vi "Drying_Process (SubVI).vi"(9 "Array 2":string[](array[string]), 10 "reference in":refnum<vi>, 11 "Array in":refnum<vi>) -> (1 "Array":string[](array[string]), 2 "Boolean":bool, 3 "empty?":bool)   [LabVIEW 2019]
uses:
  <vilib>/numeric/Random Number (Range) DBL.vi
  16b95fc4-76d9-4825-bb8f-a7daa67df2e8.vi
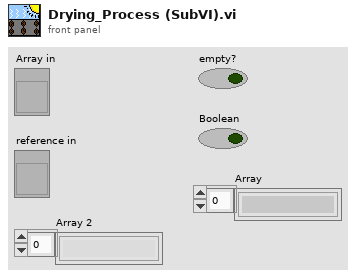
[diagram p1: front panel]
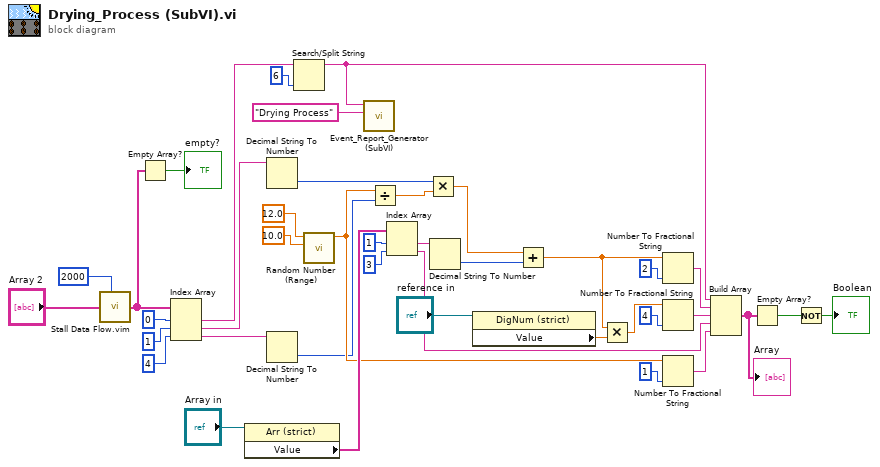
[diagram p0: block diagram]
diagram:
  n1 = call "Stall Data Flow.vim"("value in"="Array 2", "milliseconds to wait"=u32 2000) -> ("value out"=w37:string[])  [unwired: 1 out]
  n2 = Empty Array?(array=w37) -> (empty?=→"empty?":bool)
  n3 = Index Array(array=w37, index #1=0 ("index"), index #2=1 ("index"), index #3=4 ("index")) -> (element #1=w18:string, element #2=w22:string, element #3=w6:string)
  n4 = property class="Arr (strict)"(reference="Array in") -> ("Value"=w20:string[])  [unwired: 1 in, 2 out]
  n5 = Decimal String To Number(string=w22) -> (number=w3:i32)  [unwired: 2 in, 1 out]
  n6 = Decimal String To Number(string=w6) -> (number=w4:i32)  [unwired: 2 in, 1 out]
  n7 = Search/Split String(string=w18, offset (0)=6) -> (substring before match=w9:string)  [unwired: 1 in, 2 out]
  n8 = call-poly <vilib>:"Random Number (Range).vi"("lower bound (0)"=10.0, "upper bound (100)"=12.0) -> ("number"=w5:dbl)  [unwired: 9 in]
  n9 = call "Event_Report_Generator (SubVI).vi"("Process Name"="Drying Process", "Booking ID"=w9) -> ()  [unwired: 10 in]
  n10 = Divide(x=w5, y=w4) -> (x/y=w2:dbl)
  n11 = Index Array(array=w20, index #1=1 ("index"), index #2=3 ("index")) -> (element #1=w21:string, element #2=w32:string)
  n12 = Multiply(x=w3, y=w2) -> (x*y=w1:dbl)
  n13 = Decimal String To Number(string=w21) -> (number=w23:i32)  [unwired: 2 in, 1 out]
  n14 = property class="DigNum (strict)"(reference="reference in") -> ("Value"=w27:dbl)  [unwired: 1 in, 2 out]
  n15 = Add(x=w1, y=w23) -> (x+y=w26:dbl)
  n16 = Multiply(x=w26, y=w27) -> (x*y=w29:dbl)
  n17 = Number To Fractional String(number=w26, precision (6)=i16 2) -> (F-format string=w25:string)  [unwired: 2 in]
  n18 = Number To Fractional String(number=w29, precision (6)=i16 4) -> (F-format string=w30:string)  [unwired: 2 in]
  n19 = Number To Fractional String(number=w5, precision (6)=i16 1) -> (F-format string=w35:string)  [unwired: 2 in]
  n20 = Build Array(w9, w25, w30, w32, w35) -> (w7:string[])
  "Array" <- w7
  n21 = Empty Array?(array=w7) -> (empty?=w34:bool)
  n22 = Not(x=w34) -> (.not. x?=→"Boolean":bool)
